vi "Populate Tree.vi"(0 "Display State In":T1={"Hierarchy"=[], "File/Directory Path"=path "", "Relative File Paths"=[], "Hide Undefined Channels"=FALSE, "Static File Structure"=FALSE, "Filtering"={"Filtered Groups"=[], "Group Filter Mode"=enum."Exclude", "Group Filter Regex?"=FALSE, "Filtered Channels"=[], "Channel Filter Mode"=enum."Exclude", "Channel Filter Regex?"=FALSE, "Filter Time Start"=timestamp(0 s since 1904-01-01), "Filter Time End"=timestamp(0 s since 1904-01-01), "Time Filter Mode"=enum."Include", "Time Filter Enabled"=FALSE}, "File Contents Tree"=refnum, "Properties Table"=refnum, "Loading Indicator"=refnum}, 9 "Container State":T4, 11 "error in (no error)":errorcluster) -> (4 "Display State Out":T1={"Hierarchy"=[], "File/Directory Path"=path "", "Relative File Paths"=[], "Hide Undefined Channels"=FALSE, "Static File Structure"=FALSE, "Filtering"={"Filtered Groups"=[], "Group Filter Mode"=enum."Exclude", "Group Filter Regex?"=FALSE, "Filtered Channels"=[], "Channel Filter Mode"=enum."Exclude", "Channel Filter Regex?"=FALSE, "Filter Time Start"=timestamp(0 s since 1904-01-01), "Filter Time End"=timestamp(0 s since 1904-01-01), "Time Filter Mode"=enum."Include", "Time Filter Enabled"=FALSE}, "File Contents Tree"=refnum, "Properties Table"=refnum, "Loading Indicator"=refnum}, 15 "error out":errorcluster)   [LabVIEW 2017, in "XTree.xctl"]
doc: "Populates the tree according to the specified data directory, hierarchy, and filtering settings."
uses:
  <vilib>/addons/_NIFileIO/XTree/XTree.xctl
  <vilib>/_xctls/Container State.ctl
  <vilib>/addons/_NIFileIO/XTree/State.ctl
  <vilib>/addons/_NIFileIO/XTree/Controls/Filter Settings.ctl
  <vilib>/addons/_NIFileIO/XTree/Controls/Filter Mode.ctl
  <vilib>/_xctls/XControlSupport.lvlib
panel:
  # "Add Controls & Indicators that form the parameters of the method here. Hook them to the connector pane. Do not delete the controls & indicators that are already hooked to the connector pane.\n \nTo setup the parameters  for this method, right click on this item in the Project Tree & select \"Configure Method...\"."
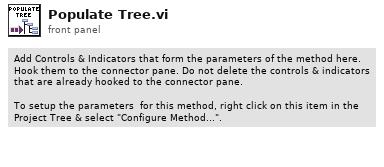
[diagram p1: front panel]
types:
  T1 = typedef "XTree.xctl/State.ctl" = cluster{"Hierarchy":string[], "File/Directory Path":path, "Relative File Paths":string[], "Hide Undefined Channels":bool, "Static File Structure":bool, "Filtering":T2, "File Contents Tree":refnum<vi>, "Properties Table":refnum<vi>, "Loading Indicator":refnum<vi>}
  T2 = typedef "XTree.xctl/Filter Settings.ctl" = cluster{"Filtered Groups":string[], "Group Filter Mode":T3, "Group Filter Regex?":bool, "Filtered Channels":string[], "Channel Filter Mode":T3, "Channel Filter Regex?":bool, "Filter Time Start":timestamp, "Filter Time End":timestamp, "Time Filter Mode":T3, "Time Filter Enabled":bool}
  T3 = typedef "XTree.xctl/Filter Mode.ctl" = enum16{"Exclude", "Include"}
  T4 = typedef "XControlSupport.lvlib/Container State.ctl" = cluster{"Indicator?":bool, "Run Mode?":bool, " Refnum":refnum<vi>}
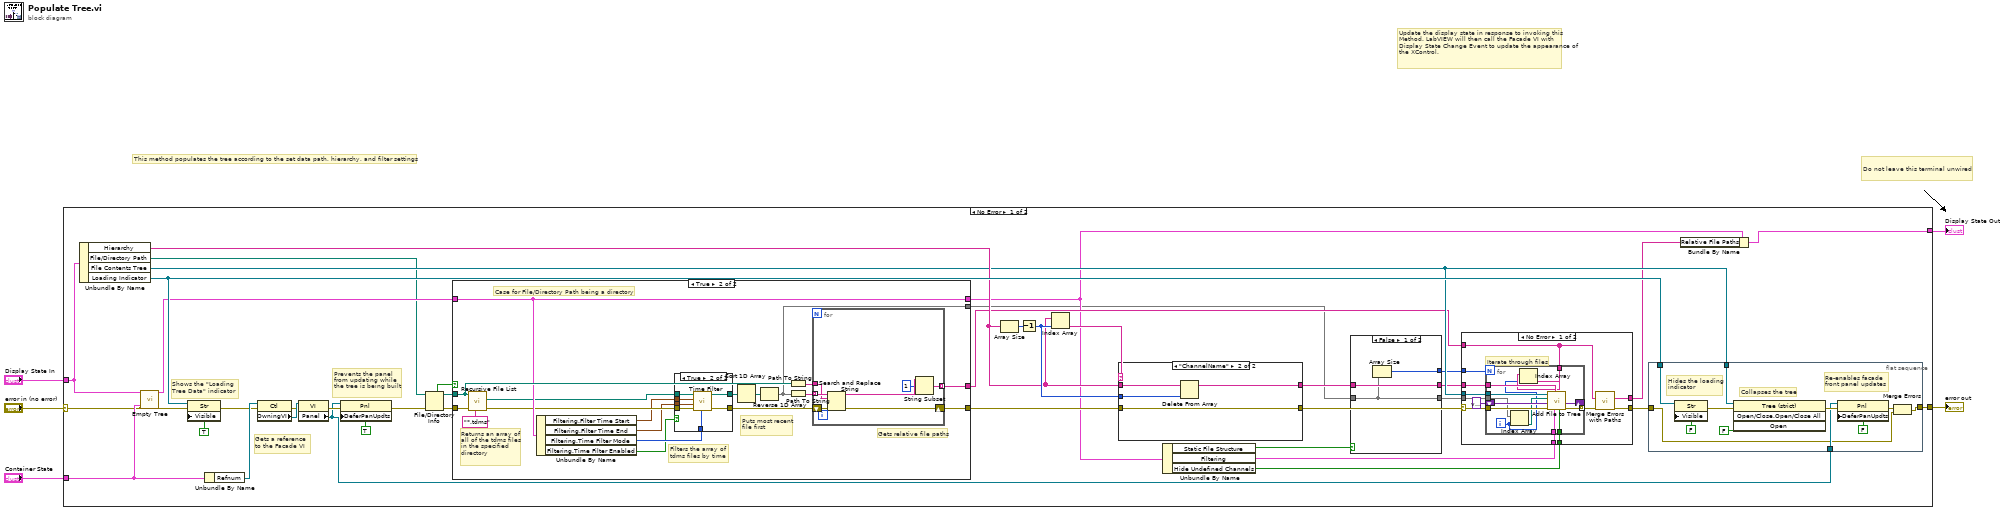
[diagram p0: block diagram]
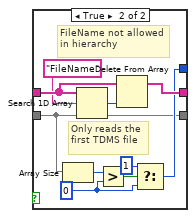
[diagram p3: hidden frame]
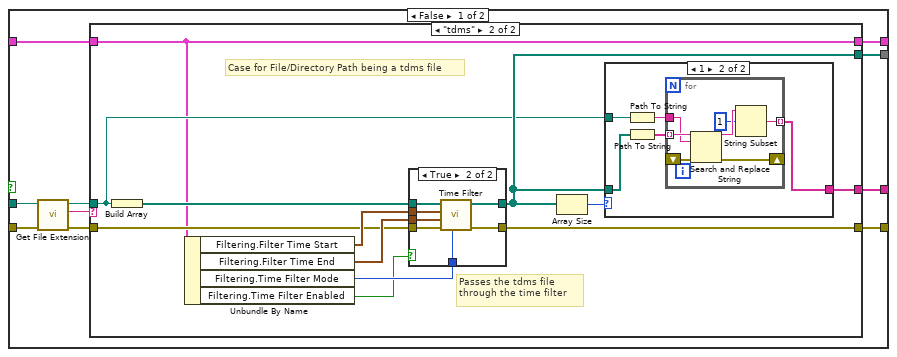
[diagram p4: hidden frame]
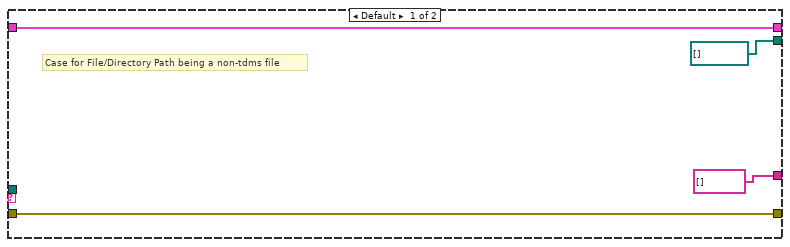
[diagram p5: hidden frame]
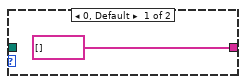
[diagram p6: hidden frame]
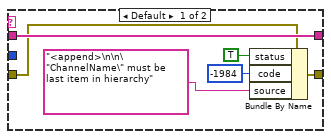
[diagram p9: hidden frame]
diagram:
  # "This method populates the tree according to the set data path, hierarchy, and filter settings"
  # "Do not leave this terminal unwired"
  # "Update the display state in response to invoking this Method. LabVIEW will then call the Facade VI with Display State Change Event to update the appearance of the XControl."
  n1 = case shown="No Error" "error in (no error)" {
    selector: "error in (no error)" -> [w31 w189]
    tunnel: [w6 w189] -> w5
    tunnel: "Display State In" -> [w28 w190]
    tunnel: [w17 w190] -> w2
    tunnel: "Container State" -> [w37 _]
    frame No Error {
      # "Prevents the panel from updating while the tree is being built"
      # "Gets a reference to the Facade VI"
      # "Shows the \"Loading Tree Data\" indicator"
      n2 = Unbundle By Name(w28) -> ("Hierarchy"=w29:string[], "File/Directory Path"=w23:path, "File Contents Tree"=w24:refnum<vi>, "Loading Indicator"=w32:refnum<vi>)
      n3 = call <vilib>:"Empty Tree.vi"("Display State In"=w28, "Container State"=w37, "error in (no error)"=w31) -> ("Display State Out"=w27:T1, "error out"=w36:errorcluster)  [unwired: 11 in]
      n4 = property class="Str"(reference=w32, error in=w36, "Visible"=TRUE) -> (error out=w35:errorcluster)  [unwired: 1 out]
      n5 = Unbundle By Name(w37) -> ("Refnum"=w39:refnum<vi>)
      n6 = property class="Ctl"(reference=w39, error in=w35) -> (error out=w33:errorcluster, "OwningVI"=w38:refnum<vi>)  [unwired: 1 out]
      n7 = property class="VI"(reference=w38, error in=w33) -> (error out=w41:errorcluster, "Panel"=w7:refnum<vi>)  [unwired: 1 out]
      n8 = property class="Pnl"(reference=w7, error in=w41, "DeferPanUpdts"=TRUE ("Defer Panel Updates")) -> (error out=w22:errorcluster)  [unwired: 1 out]
      n9 = File/Directory Info(path=w23, error in=w22) -> (path out=w21:path, directory=w20:bool, error out=w19:errorcluster)  [unwired: 4 out]
      n10 = case shown="True" w20 {
        tunnel: w21 -> [w100 w158]
        tunnel: w27 -> [w104 w153]
        tunnel: [w97 w153] -> w15
        tunnel: w19 -> [w102 w161]
        tunnel: [w105 w155] -> w30
        tunnel: [w103 w156] -> w10
        tunnel: [w106 w154] -> w16
        frame False {
          n11 = call <vilib>:"Get File Extension.vi"("error in (no error)"=w102, "file"=w100) -> ("error out"=w101:errorcluster, "lowercase file extension"=w98:string, "dup file"=w99:path)  [unwired: 5 in, 2 out]
          n12 = case shown="\"tdms\"" w98 {
            tunnel: [string[] [] w122] -> w106
            tunnel: [w108 w117] -> w105
            tunnel: w104 -> [w107 w111]
            tunnel: [path[] [] w113] -> w103
            tunnel: w101 -> [w108 w114]
            tunnel: w99 -> [_ w112]
            tunnel: [w107 w111] -> w97
            frame Default {
              # "Case for File/Directory Path being a non-tdms file"
            }
            frame "tdms" {
              # "Passes the tdms file through the time filter"
              # "Case for File/Directory Path being a tdms file"
              n13 = Build Array(w112) -> (w116:path[])
              n14 = Unbundle By Name(w111) -> ("Filtering.Filter Time Start"=w121:timestamp, "Filtering.Filter Time End"=w120:timestamp, "Filtering.Time Filter Mode"=w119:T3, "Filtering.Time Filter Enabled"=w118:bool)
              n15 = case shown="True" w118 {
                tunnel: w114 -> [w136 w144]
                tunnel: [w136 w143] -> w117
                tunnel: [w137 w142] -> w113
                tunnel: w116 -> [w137 w141]
                tunnel: w121 -> [_ w140]
                tunnel: w120 -> [_ w139]
                tunnel: w119 -> [_ w138]
                frame False {
                }
                frame True {
                  n16 = call <vilib>:"Time Filter.vi"("Filter Mode"=w138, "error in (no error)"=w144, "Filter Time End"=w139, "Filter Time Start"=w140, "TDMS Paths In"=w141) -> ("error out"=w143:errorcluster, "TDMS Paths Out"=w142:path[])  [unwired: 5 in]
                }
              }
              n17 = Array Size(array=w113) -> (size(s)=w115:i32)
              n18 = case shown="1" w115 {
                tunnel: [string[] [] w124] -> w122
                tunnel: w113 -> [_ w125]
                tunnel: w112 -> [_ w126]
                frame 0, Default {
                }
                frame 1 {
                  n19 = Path To String(path=w126) -> (string=w127:string)
                  n20 = Path To String(path=w125) -> (string=w128:string[])
                  n21 = for {
                    tunnel: w128 -> [w135] mode=indexing
                    tunnel: w127 -> [w134]
                    shift-right: [w129] -> _
                    shift-left: _ -> [w133]
                    tunnel: [w130] -> w124 mode=indexing
                    n22 = Search and Replace String(input string=w135, search string=w134, error in=w133) -> (result string=w132:string, error out=w129:errorcluster)  [unwired: 5 in, 2 out]
                    n23 = String Subset(string=w132, offset (0)=1) -> (substring=w130:string)  [unwired: 1 in]
                  }
                }
              }
            }
          }
        }
        frame True {
          # "Returns an array of all of the tdms files in the specified directory"
          # "Filters the array of tdms files by time"
          # "Case for File/Directory Path being a directory"
          # "Gets relative file paths"
          # "Puts most recent file first"
          n24 = call <vilib>:"Recursive File List.vi"("pattern"="*.tdms", "error in (no error)"=w161, "Folder Path"=w158) -> ("error out"=w152:errorcluster, "All Files in Dir"=w149:path[])  [unwired: 4 in, 3 out]
          n25 = Unbundle By Name(w153) -> ("Filtering.Filter Time Start"=w148:timestamp, "Filtering.Filter Time End"=w147:timestamp, "Filtering.Time Filter Mode"=w146:T3, "Filtering.Time Filter Enabled"=w145:bool)
          n26 = case shown="True" w145 {
            tunnel: w152 -> [w163 w171]
            tunnel: [w163 w170] -> w151
            tunnel: [w164 w169] -> w150
            tunnel: w149 -> [w164 w168]
            tunnel: w148 -> [_ w167]
            tunnel: w147 -> [_ w166]
            tunnel: w146 -> [_ w165]
            frame False {
            }
            frame True {
              n27 = call <vilib>:"Time Filter.vi"("Filter Mode"=w165, "error in (no error)"=w171, "Filter Time End"=w166, "Filter Time Start"=w167, "TDMS Paths In"=w168) -> ("error out"=w170:errorcluster, "TDMS Paths Out"=w169:path[])  [unwired: 5 in]
            }
          }
          n28 = Sort 1D Array(array=w150) -> (sorted array=w160:path[])
          n29 = Reverse 1D Array(array=w160) -> (reversed array=w156:path[])
          n30 = Path To String(path=w158) -> (string=w157:string)
          n31 = Path To String(path=w156) -> (string=w159:string[])
          n32 = for {
            tunnel: w159 -> [w178] mode=indexing
            tunnel: w157 -> [w177]
            shift-right: [w172] -> w155
            shift-left: w151 -> [w176]
            tunnel: [w173] -> w154 mode=indexing
            n33 = Search and Replace String(input string=w178, search string=w177, error in=w176) -> (result string=w175:string, error out=w172:errorcluster)  [unwired: 5 in, 2 out]
            n34 = String Subset(string=w175, offset (0)=1) -> (substring=w173:string)  [unwired: 1 in]
          }
        }
      }
      n35 = Array Size(array=w29) -> (size(s)=w45:i32)
      n36 = Decrement(x=w45) -> (x-1=w43:i32)
      n37 = Index Array(array=w29, index=w43) -> (element=w44:string)
      n38 = case shown="\"ChannelName\"" w44 {
        tunnel: [w182 w188] -> w8
        tunnel: w30 -> [w183 w188]
        tunnel: w29 -> [w184 w187]
        tunnel: w43 -> [_ w186]
        tunnel: [w184 w185] -> w42
        frame Default {
          n39 = Bundle By Name(cluster=w183, "status"=TRUE, "code"=-1984, "source"="<append>\n\n\"ChannelName\" must be last item in hierarchy") -> (w182:errorcluster)
        }
        frame "ChannelName" {
          n40 = Delete From Array(array=w187, index=w186) -> (array with subset deleted=w185:string[])  [unwired: 1 in, 1 out]
        }
      }
      n41 = Unbundle By Name(w15) -> ("Static File Structure"=w11:bool, "Filtering"=w26:T2, "Hide Undefined Channels"=w25:bool)
      n42 = case shown="False" w11 {
        tunnel: w42 -> [w74 w85]
        tunnel: [w75 w78] -> w13
        tunnel: [w74 w82] -> w12
        tunnel: w10 -> [w73 w77]
        tunnel: [w73 w77] -> w9
        frame False {
          n43 = Array Size(array=w73) -> (size(s)=w75:i32)
        }
        frame True {
          w79 = 0 ("y")
          # "Only reads the first TDMS file"
          # "FileName not allowed in hierarchy"
          n44 = Array Size(array=w77) -> (size(s)=w81:i32)
          n45 = Search 1D Array(1D array=w85, element="FileName") -> (index of element=w83:i32)  [unwired: 1 in]
          n46 = Greater?(x=w81, y=w79) -> (0:w80:bool)
          n47 = Delete From Array(array=w85, index=w83) -> (array with subset deleted=w82:string[])  [unwired: 1 in, 1 out]
          n48 = Select(t=1, s=w80, f=w79) -> (s? t:f=w78:i32)
        }
      }
      n49 = case shown="No Error" w8 {
        selector: w8 -> [w46 w71]
        tunnel: w26 -> [w57 _]
        tunnel: w25 -> [w56 _]
        tunnel: w24 -> [w55 _]
        tunnel: [w53 w71] -> w18
        tunnel: w16 -> [w47 w72]
        tunnel: [w52 w72] -> w14
        tunnel: w13 -> [w50 _]
        tunnel: w12 -> [w49 _]
        tunnel: w9 -> [w48 _]
        frame No Error {
          # "Iterate through files"
          n50 = for {
            N: w50 -> [_]
            tunnel: w49 -> [w69]
            tunnel: w48 -> [w62]
            shift-right: [w66] -> _
            shift-left: variant ("Tree Items Created Out") -> [w68]
            tunnel: w55 -> [w67]
            tunnel: w57 -> [w64]
            tunnel: w56 -> [w63]
            tunnel: w47 -> [w60]
            tunnel: w46 -> [w70]
            tunnel: [w65] -> w54 mode=indexing
            i -> [w59]
            n51 = Index Array(array=w62, index=w59) -> (element=w61:path)
            n52 = Index Array(array=w60, index=w59) -> (element=w58:string)
            n53 = call <vilib>:"Add File to Tree.vi"("Hide Undefined Channels"=w63, "Relative File Path"=w58, "Filter Settings"=w64, "Hierarchy"=w69, "error in (no error)"=w70, "Tree Items Created In"=w68, "File Path"=w61, "TreeControl in"=w67) -> ("error out"=w65:errorcluster, "Tree Items Created Out"=w66:variant)  [unwired: 2 in]
          }
          n54 = call <vilib>:"Merge Errors with Paths.vi"("Errors"=w54, "Relative File Paths In"=w47) -> ("error out"=w53:errorcluster, "Relative File Paths Out"=w52:string[])  [unwired: 8 in]
        }
        frame Error {
        }
      }
      n55 = flat-sequence {
        tunnel: w32 -> [w94]
        tunnel: w24 -> [w93]
        tunnel: w18 -> [w88]
        tunnel: w7 -> [w90]
        tunnel: [w86] -> w6
        frame #0 {
          # "Re-enables facade front panel updates"
          # "Hides the loading indicator"
          # "Collapses the tree"
          n56 = property class="Str"(reference=w94, "Visible"=FALSE) -> (error out=w92:errorcluster)  [unwired: 1 in, 1 out]
          n57 = invoke class="Tree (strict)" method="Open/Close.Open/Close All"(reference=w93, error in=w92, "Open"=FALSE ("Open?")) -> (error out=w91:errorcluster)  [unwired: 1 in, 3 out]
          n58 = property class="Pnl"(reference=w90, error in=w91, "DeferPanUpdts"=FALSE ("Defer Panel Updates")) -> (error out=w87:errorcluster)  [unwired: 1 out]
          n59 = Merge Errors(w87, w88) -> (w86:errorcluster)
        }
      }
      n60 = Bundle By Name(cluster=w15, "Relative File Paths"=w14) -> (w17:T1)
    }
    frame Error {
    }
  }
  "error out" <- w5
  "Display State Out" <- w2
